vi "Set message.vi"(10 "WampMessage MsgPack":refnum<class "WampMessage MsgPack.lvclass">, 11 "AbortHandler MsgPack in":refnum<class "AbortHandler MsgPack.lvclass">) -> (3 "AbortHandler MsgPack out":refnum<class "AbortHandler MsgPack.lvclass">)   [LabVIEW 2020, in "wamplv.lvlib" / "AbortHandler MsgPack.lvclass"]
uses:
  AbortHandler MsgPack.lvclass
  AbortHandler MsgPack.lvclass/AbortHandler MsgPack.ctl
  SerialisedMessages/MsgPackMessage/WampMessage MsgPack.lvclass
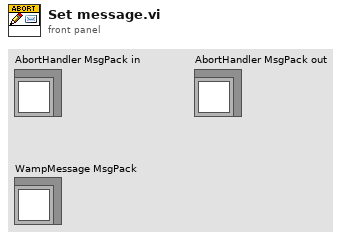
[diagram p1: front panel]
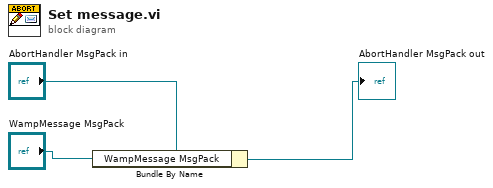
[diagram p0: block diagram]
diagram:
  n1 = Bundle By Name(cluster="AbortHandler MsgPack in", "WampMessage MsgPack"="WampMessage MsgPack") -> (→"AbortHandler MsgPack out":refnum<class "AbortHandler MsgPack.lvclass">)
